vi "Button Pitch Test.vi"() -> ()   [LabVIEW 2026]
uses:
  <vilib>/rvi/Emulation/niFpgaGetClockAttributes.vi
  <vilib>/rvi/Emulation/niFpgaSctlEmulationGetInTimedLoop.vi
  <vilib>/rvi/Emulation/niFpgaEmulationReportErrorSimple.vi
  <vilib>/rvi/eio/common/nirviEmuTemplateMethod_errors.vi
  <vilib>/rvi/Emulation/niFpgaCriticalErrorInLSC.vi
  <vilib>/eio/EIONode/EIONode.xnode
panel:
  in  "Count(uSec)":u32 caption="Sound Duration"
  in  "Duty Cycle On":u16 caption="Duty Cycle\n (How long stays on)"
  out "Numeric":i32
  in  "Duty Cycle Off":u16 caption="Duty Cycle\n (How long stays on)"
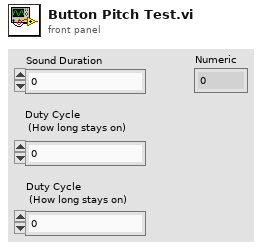
[diagram p1: front panel]
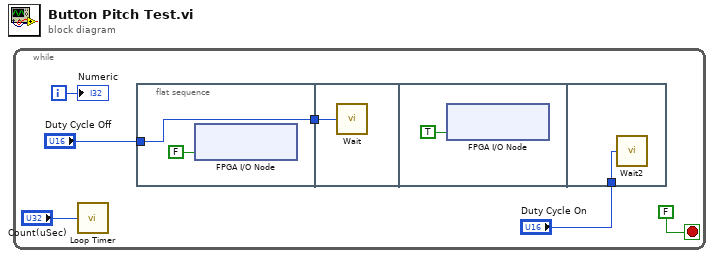
[diagram p0: block diagram]
diagram:
  n1 = while {
    i -> [w4]
    stop <- FALSE ("stop") stop-if-true
    n2 = call "Loop Timer"("Count(uSec)"="Count(uSec)") -> ()  [unwired: 1 out]
    n3 = flat-sequence {
      tunnel: "Duty Cycle Off" -> [w8]
      tunnel: [w8] -> w5
      tunnel: w5 -> [w9]
      tunnel: "Duty Cycle On" -> [w11]
      frame #0 {
        n4 = xnode "FPGA I/O Node"("Mod1/DO0"=FALSE) -> ()  [unwired: 1 in, 1 out]
      }
      frame #1 {
        n5 = call "Wait"("Count(uSec)"=w9) -> ()  [unwired: 1 out]
      }
      frame #2 {
        n6 = xnode "FPGA I/O Node"("Mod1/DO0"=TRUE) -> ()  [unwired: 1 in, 1 out]
      }
      frame #3 {
        n7 = call "Wait2"("Count(uSec)"=w11) -> ()  [unwired: 1 out]
      }
    }
    "Numeric" <- w4
  }
